vi "inversa.vi"(8 "delta theta":dbl, 10 "theta":dbl) -> (2 "dt":dbl)   [LabVIEW 2018]
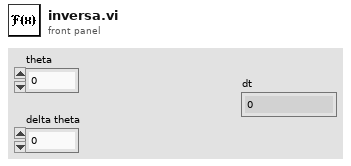
[diagram p1: front panel]
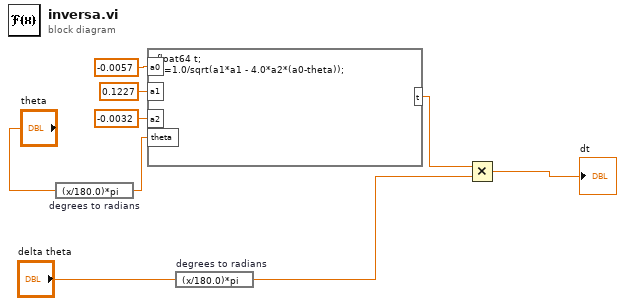
[diagram p0: block diagram]
diagram:
  n1 = expression code="(x/180.0)*pi" "degrees to radians"("theta") -> (w4:dbl)
  n2 = formula code="float64 t;\nt =1.0/sqrt(a1*a1 - 4.0*a2*(a0-theta));"("a0"=-0.0057 ("input variable"), "a1"=0.1227 ("input variable"), "a2"=-0.0032 ("input variable"), "theta"=w4) -> ("t"=w6:dbl)
  n3 = expression code="(x/180.0)*pi" "degrees to radians"("delta theta") -> (w2:dbl)
  n4 = Multiply(x=w6, y=w2) -> (x*y=→"dt":dbl)
